vi "_Create Base Log Folder.vi"(7 "Application Name":string, 8 "Error In":errorcluster, 11 "Root Folder":path) -> (0 "Error Out":errorcluster, 3 "Base Log Folder":path)   [LabVIEW 2014, in "Logger.lvlib"]
uses:
  Logger.lvlib
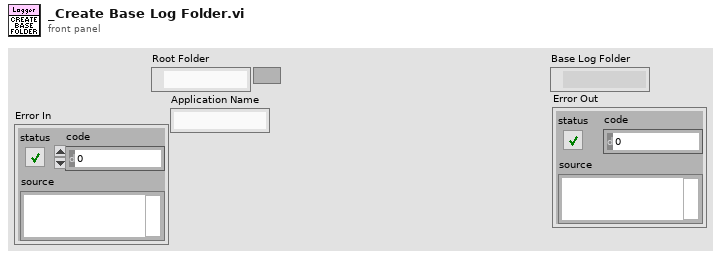
[diagram p1: front panel]
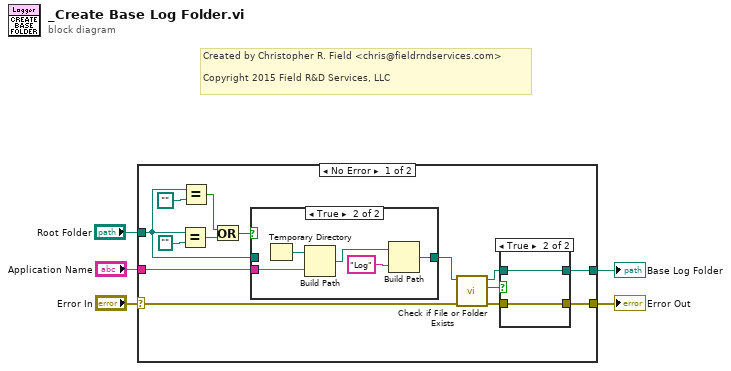
[diagram p0: block diagram]
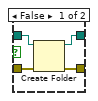
[diagram p2: hidden frame]
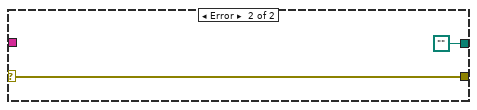
[diagram p4: hidden frame]
diagram:
  # "Created by Christopher R. Field <chris@fieldrndservices.com>\n\nCopyright 2015 Field R&D Services, LLC"
  n1 = case shown="No Error" "Error In" {
    selector: "Error In" -> [w11 w33]
    tunnel: "Root Folder" -> [w14 _]
    tunnel: "Application Name" -> [w13 _]
    tunnel: [w7 path ""] -> w2
    tunnel: [w6 w33] -> w1
    frame No Error {
      n2 = Equal?(x=w14, y=path "") -> (x = y?=w16:bool)
      n3 = Equal?(x=w14, y=path "") -> (x = y?=w17:bool)
      n4 = Or(x=w17, y=w16) -> (x .or. y?=w15:bool)
      n5 = case shown="True" w15 {
        tunnel: [w26 w29] -> w12
        tunnel: w14 -> [w26 _]
        tunnel: w13 -> [_ w27]
        frame False {
        }
        frame True {
          n6 = Temporary Directory() -> (w31:path)
          n7 = Build Path(base path=w31, name or relative path=w27) -> (appended path=w28:path)
          n8 = Build Path(base path=w28, name or relative path="Log") -> (appended path=w29:path)
        }
      }
      n9 = call <vilib>:"Check if File or Folder Exists.vi"("error in (no error)"=w11, "path"=w12) -> ("error out"=w8:errorcluster, "file or folder exists?"=w10:bool, "dup path"=w9:path)  [unwired: 7 in]
      n10 = case shown="True" w10 {
        tunnel: w9 -> [w23 w25]
        tunnel: w8 -> [w22 w24]
        tunnel: [w21 w25] -> w7
        tunnel: [w20 w24] -> w6
        frame False {
          n11 = Create Folder(path (use dialog)=w23, error in=w22) -> (created path=w21:path, error out=w20:errorcluster)  [unwired: 1 in, 1 out]
        }
        frame True {
        }
      }
    }
    frame Error {
    }
  }
  "Base Log Folder" <- w2
  "Error Out" <- w1
